vi "Amplitud.vi"(8 "error in (no error)":errorcluster, 10 "Numeric":dbl, 11 "Generador de Funciones in":refnum<class "Generador de Funciones.lvclass">) -> (0 "error out":errorcluster, 3 "Generador de Funciones out":refnum<class "Generador de Funciones.lvclass">)   [LabVIEW 2020, in "Generador de Funciones.lvlib" / "Generador de Funciones.lvclass"]
uses:
  Generador de Funciones.lvclass
  Generador de Funciones.lvclass/Generador de Funciones.ctl
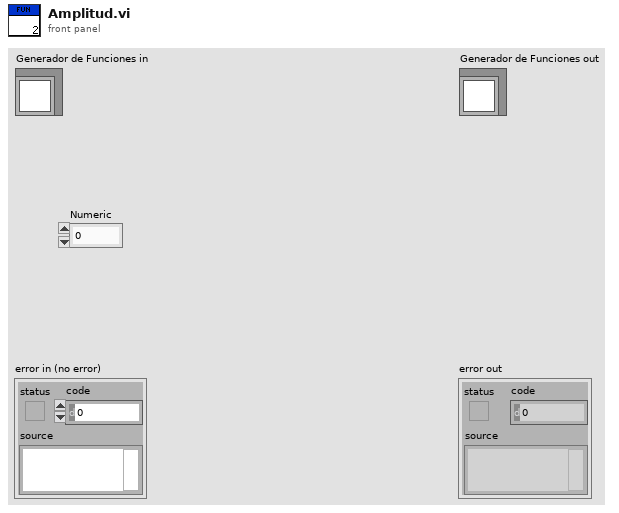
[diagram p1: front panel]
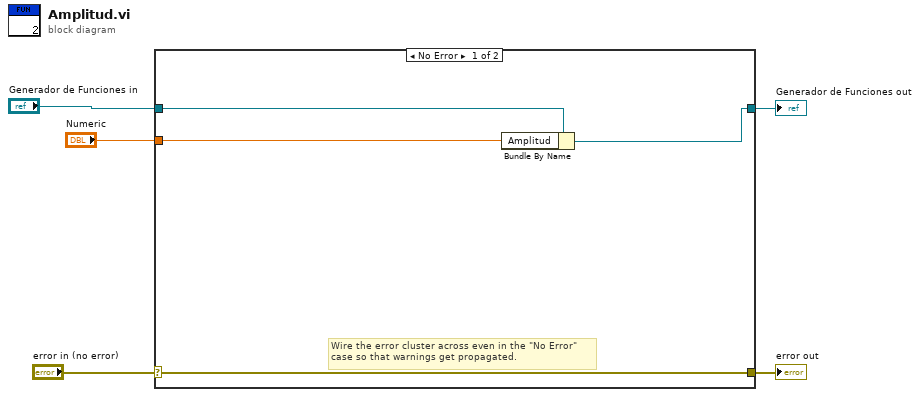
[diagram p0: block diagram]
diagram:
  n1 = case shown="No Error" "error in (no error)" {
    selector: "error in (no error)" -> [w9 w11]
    tunnel: [w9 w11] -> w4
    tunnel: [w7 w10] -> w2
    tunnel: "Generador de Funciones in" -> [w8 w10]
    tunnel: "Numeric" -> [w6 _]
    frame No Error {
      # "Wire the error cluster across even in the \"No Error\"\ncase so that warnings get propagated."
      n2 = Bundle By Name(cluster=w8, "Amplitud"=w6) -> (w7:refnum<class "Generador de Funciones.lvclass">)
    }
    frame Error {
    }
  }
  "error out" <- w4
  "Generador de Funciones out" <- w2
